vi "set handle.vi"(8 "error in (no error)":errorcluster, 10 "handle":dbl, 11 "someclass in":refnum<class "someclass.lvclass">) -> (0 "error out":errorcluster, 3 "someclass out":refnum<class "someclass.lvclass">)   [LabVIEW 2023, in "somelib.lvlib" / "someclass.lvclass"]
uses:
  someclass.lvclass
  someclass.lvclass/someclass.ctl
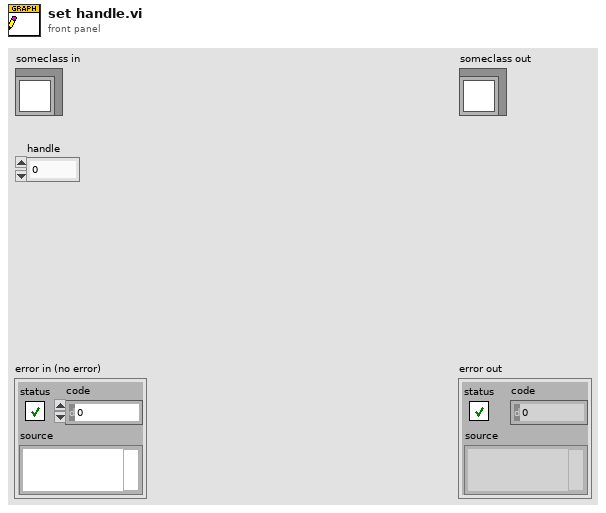
[diagram p1: front panel]
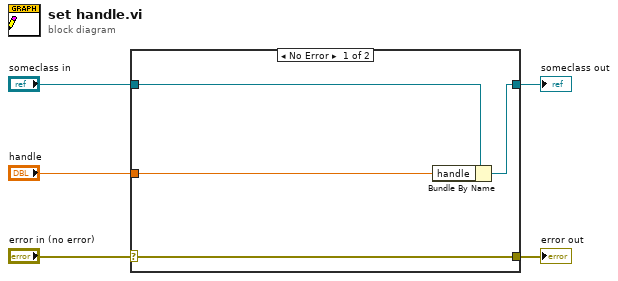
[diagram p0: block diagram]
diagram:
  n1 = case shown="No Error" "error in (no error)" {
    selector: "error in (no error)" -> [w9 w10]
    tunnel: [w9 w10] -> w4
    tunnel: [w7 w11] -> w2
    tunnel: "someclass in" -> [w8 w11]
    tunnel: "handle" -> [w6 _]
    frame No Error {
      n2 = Bundle By Name(cluster=w8, "handle"=w6) -> (w7:refnum<class "someclass.lvclass">)
    }
    frame Error {
    }
  }
  "error out" <- w4
  "someclass out" <- w2
